vi "acquisition_play.vi"(3 "error in":errorcluster, 4 "number of samples per channel":i32=-1, 5 "task/channels in":refnum<k21>) -> (0 "error out":errorcluster, 1 "WFM":waveform(dbl)[](array[waveform]), 2 "task out":refnum<k21>)   [LabVIEW 2017]
uses:
  <vilib>/DAQmx/read.llb/DAQmx Read (Analog 1D Wfm NChan NSamp).vi
  <vilib>/DAQmx/miscellaneous.llb/DAQmx Fill In Error Info.vi
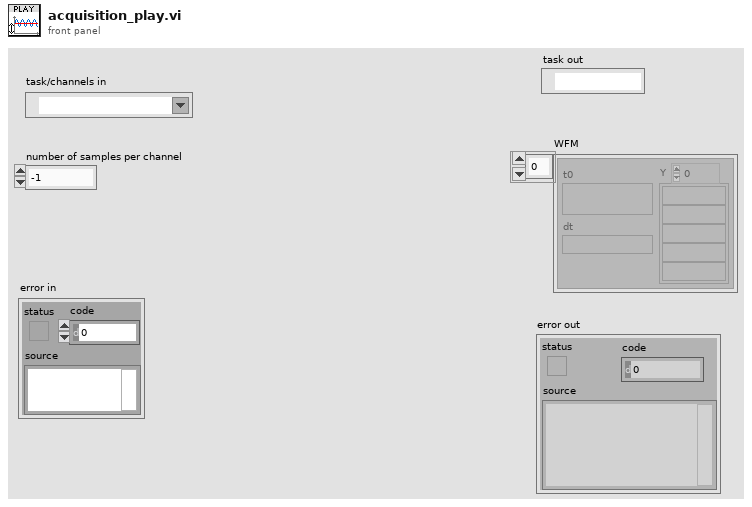
[diagram p1: front panel]
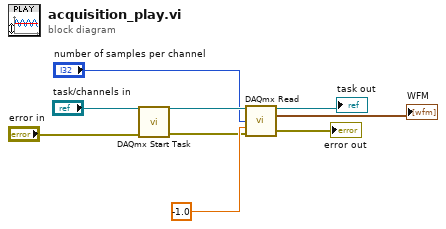
[diagram p0: block diagram]
diagram:
  n1 = call <vilib>:"DAQmx Start Task.vi"("task/channels in"="task/channels in", "error in"="error in") -> ("task out"=w4:refnum<k21>, "error out"=w3:errorcluster)  [unwired: 12 in]
  n2 = call-poly <vilib>:"DAQmx Read.vi"("task/channels in"=w4, "number of samples per channel"="number of samples per channel", "timeout"=-1.0, "error in"=w3) -> ("task out"=→"task out":refnum<k21>, "data"=→"WFM":waveform(dbl)[], "error out"=→"error out":errorcluster)  [unwired: 9 in]
